vi "Create Message Transport.vi"(7 "Transport Name":string, 8 "error in":errorcluster, 10 "Transport Payload type":refnum<class "IMessagePayload.lvclass">, 11 "UserEventMessageTransport":refnum<class "UserEventMessageTransport.lvclass">) -> (0 "error out":errorcluster, 3 "UserEventMessageTransport":refnum<class "UserEventMessageTransport.lvclass">)   [LabVIEW 2016, in "UserEventMessageTransport.lvclass"]
uses:
  UserEventMessageTransport.lvclass
  IMessagePayload/IMessagePayload.lvclass
panel:
  # "INPUTS"
  # "OUTPUTS"
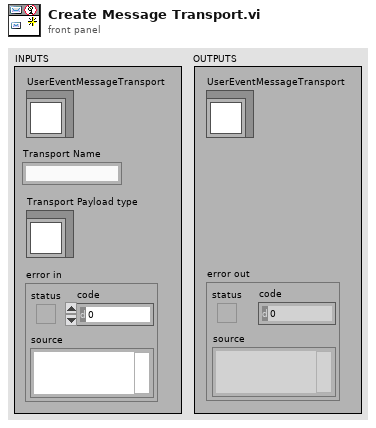
[diagram p1: front panel]
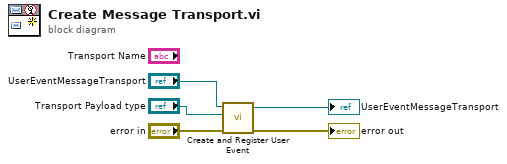
[diagram p0: block diagram]
diagram:
  n1 = call "Create and Register User Event.vi"("error in"="error in", "Payload Data Type"="Transport Payload type", "UserEventMessageTransport"="UserEventMessageTransport") -> ("error out"=→"error out":errorcluster, "UserEventMessageTransport"=→"UserEventMessageTransport":refnum<class "UserEventMessageTransport.lvclass">)  [unwired: 7 in]
